vi "LVClass_DataServer SetImage.vi"(0 "DataServer in":refnum<class "DataServer.lvclass">, 5 "name":string, 7 "Image in":refnum<class "Image.lvclass">, 11 "error in (no error)":errorcluster) -> (4 "DataServer out":refnum<class "DataServer.lvclass">, 8 "Image (dup)":refnum<class "Image.lvclass">, 15 "error out":errorcluster)   [LabVIEW 2020, in "DataServer.lvclass"]
doc: "Set data corresponding to /p name.\n\n<B>serverIn</B> : Server object.\n<B>serverOut</B> : Server object.\n<B>name</B> : Data name\n<B>data</B> : Image object."
uses:
  DataServer.lvclass
  Image.lvclass
  DataServer.lvclass/DataServer.ctl
  LVClass_Image Read Image.vi
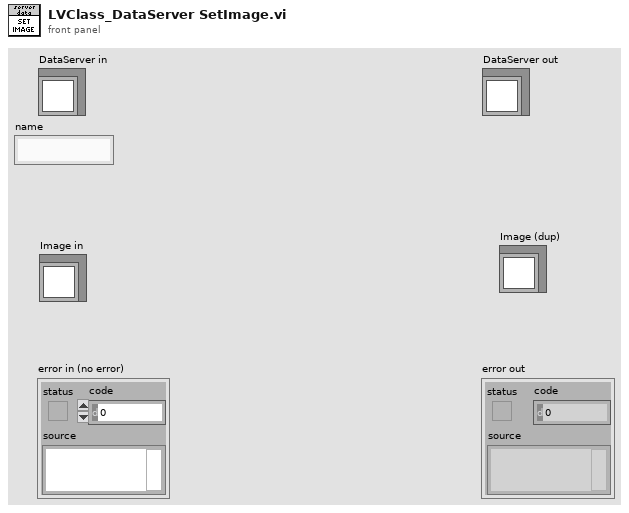
[diagram p1: front panel]
types:
  T1 = typedef "Struct_Image.ctl" = cluster{"Image_Handler":T2, "Number of bits":T3, "ImageSize":T4}
  T2 = typedef "ClassID.ctl" = i64
  T3 = typedef "Data alignment enum.ctl" = enum16{"8", "16", "32"}
  T4 = typedef "Point2D.ctl" = cluster{"X":u32, "Y":u32}
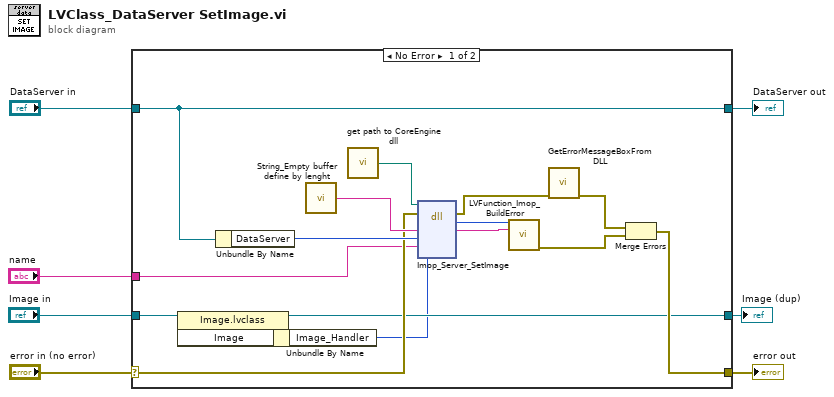
[diagram p0: block diagram]
diagram:
  n1 = case shown="No Error" "error in (no error)" {
    selector: "error in (no error)" -> [w14 w26]
    tunnel: [w13 w26] -> w6
    tunnel: [w15 w25] -> w4
    tunnel: "DataServer in" -> [w15 w25]
    tunnel: "Image in" -> [w12 w24]
    tunnel: [w10 w24] -> w2
    tunnel: "name" -> [w9 _]
    frame No Error {
      n2 = property class="Image.lvclass"(reference=w12) -> (reference out=w10:refnum<class "Image.lvclass">, "Image"=w11:T1)  [unwired: 1 in, 1 out]
      n3 = Unbundle By Name(w15) -> ("DataServer"=w21:T2)
      n4 = Unbundle By Name(w11) -> ("Image_Handler"=w8:T2)
      n5 = call "String_Empty buffer define by lenght.vi"() -> ("Empty buffer"=w18:string)  [unwired: 1 in]
      n6 = call "get path to CoreEngine dll.vi"() -> ("path to wavekit library"=w19:path)  [unwired: 14 in, 1 out]
      n7 = dll-call lib="D:/soft/HASO_v3/SVN_trunk/ImOpCoreEngine4_LV2011/DLLs/c_interface_vc100.dll" fn="Imop_Server_SetImage"(path in=w19, error in=w14, "message"=w18, "server"=w21, "name"=w9, "data"=w8) -> (error out=w20:errorcluster, "return type"=w16:i32, "message"=w17:string)  [unwired: 4 in, 1 out]
      n8 = call "LVFunction_Imop_BuildError.vi"("code"=w16, "String to Prepend to source (\"\")"=w17) -> ("error out"=w23:errorcluster)  [unwired: 13 in]
      n9 = call "GetErrorMessageBoxFromDLL.vi"("error IN"=w20) -> ("error OUT"=w22:errorcluster)  [unwired: 10 in]
      n10 = Merge Errors(w22, w23) -> (w13:errorcluster)
    }
    frame Error {
    }
  }
  "error out" <- w6
  "DataServer out" <- w4
  "Image (dup)" <- w2
